vi "Read Server RPC Methods.vi"(8 "error in (no error)":errorcluster, 11 "gRPC service in":refnum<class "ExamplePluginOOBService.lvclass">) -> (0 "error out":errorcluster, 2 "Server RPC Methods":T1, 3 "gRPC service out":refnum<class "ExamplePluginOOBService.lvclass">)   [LabVIEW 2025, in "ExamplePluginOOBService_server.lvlib" / "ExamplePluginOOBService.lvclass"]
uses:
  ExamplePluginOOBService.lvclass
  typeDefs/Server gRPC UEs.ctl
  <vilib>/gRPC/LabVIEW gRPC Library/Server API/typeDefs/gRPCId Cluster.ctl
  <vilib>/gRPC/LabVIEW gRPC Library/Shared/grpcId.ctl
  ExamplePluginOOBService.lvclass/ExamplePluginOOBService.ctl
  <vilib>/gRPC/LabVIEW gRPC Library/grpc-lvsupport-release.lvlib
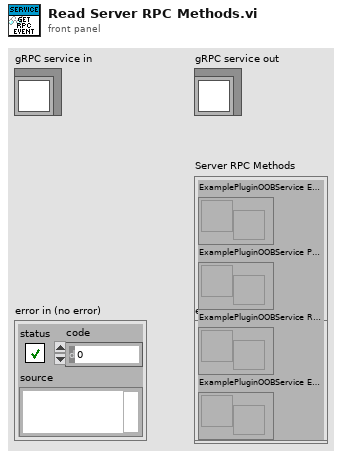
[diagram p1: front panel]
types:
  T1 = typedef "ExamplePluginOOBService_server.lvlib/ExamplePluginOOBService.lvclass/Server gRPC UEs.ctl" = cluster{"ExamplePluginOOBService Execute gRPC UE":refnum<user-event>, "ExamplePluginOOBService Pause gRPC UE":refnum<user-event>, "ExamplePluginOOBService Resume gRPC UE":refnum<user-event>, "ExamplePluginOOBService Export gRPC UE":refnum<user-event>}
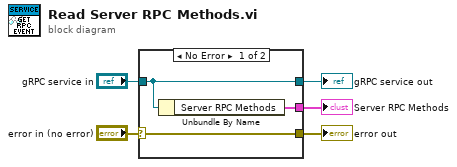
[diagram p0: block diagram]
diagram:
  n1 = case shown="No Error" "error in (no error)" {
    selector: "error in (no error)" -> [w8 w9]
    tunnel: [w8 w9] -> w4
    tunnel: [w7 w10] -> w2
    tunnel: "gRPC service in" -> [w7 w10]
    tunnel: [w6 _] -> w1
    frame No Error {
      n2 = Unbundle By Name(w7) -> ("Server RPC Methods"=w6:T1)
    }
    frame Error {
    }
  }
  "error out" <- w4
  "gRPC service out" <- w2
  "Server RPC Methods" <- w1
